vi "toggle_drain_valve.vi"(1 "set_drain_valve":bool) -> (0 "current_drain_valve_state":bool)   [LabVIEW 2018]
uses:
  <vilib>/rvi/eio/common/nirviEmuTemplateMethod_errors.vi
  <vilib>/eio/EIONode/EIONode.xnode
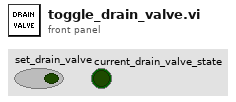
[diagram p1: front panel]
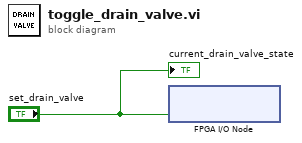
[diagram p0: block diagram]
diagram:
  n1 = xnode "FPGA I/O Node"("Mod2/DIO11"="set_drain_valve") -> ()  [unwired: 1 in, 1 out]
  "current_drain_valve_state" <- "set_drain_valve"
